vi "Read LakeShore Settings.vi"(8 "error in (no error)":errorcluster, 11 "VISA resource name":refnum<visa-resource-name>) -> (0 "error out":errorcluster, 1 "Heater level":dbl, 2 "Heater mode":T1(ring), 3 "VISA resource name out":refnum<visa-resource-name>, 4 "PID":cluster{"P":dbl, "I":dbl, "D":dbl}, 5 "Hater range":dbl, 7 "Set point":dbl)   [LabVIEW 2015]
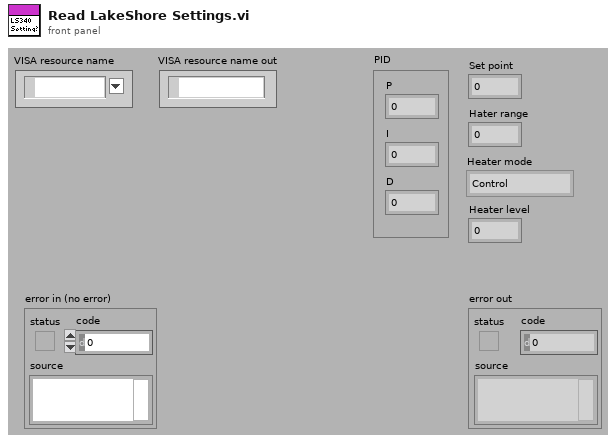
[diagram p1: front panel]
types:
  T1 = enum16{"Control", "Monitor", "Manual Heat", "Controller is in OFF mode", "Autotune is in progress"}
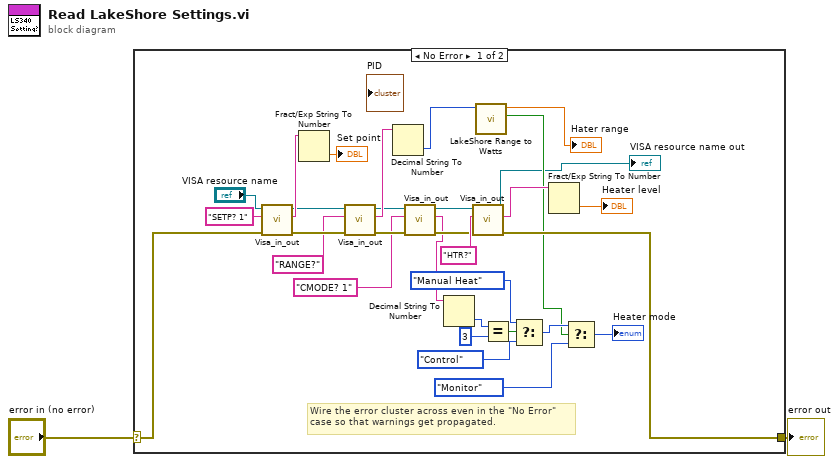
[diagram p0: block diagram]
diagram:
  n1 = case shown="No Error" "error in (no error)" {
    selector: "error in (no error)" -> [w4 w34]
    tunnel: [w17 w34] -> w1
    frame No Error {
      # "Wire the error cluster across even in the \"No Error\"\ncase so that warnings get propagated."
      n2 = call "Visa_in_out.vi"("error in (no error)"=w4, "write buffer"="SETP? 1", "VISA resource name"="VISA resource name") -> ("error out"=w30:errorcluster, "read buffer"=w32:string, "VISA resource name out"=w29:refnum<visa-resource-name>)  [unwired: 1 in, 5 out]
      n3 = Fract/Exp String To Number(string=w32) -> (number=→"Set point":dbl)  [unwired: 4 out]
      n4 = call "Visa_in_out.vi"("error in (no error)"=w30, "write buffer"="RANGE?", "VISA resource name"=w29) -> ("error out"=w19:errorcluster, "read buffer"=w27:string, "VISA resource name out"=w21:refnum<visa-resource-name>)  [unwired: 1 in, 5 out]
      n5 = Decimal String To Number(string=w27) -> (number=w26:i32)  [unwired: 3 out]
      n6 = call "Visa_in_out.vi"("error in (no error)"=w19, "write buffer"="CMODE? 1", "VISA resource name"=w21) -> ("error out"=w18:errorcluster, "read buffer"=w15:string, "VISA resource name out"=w20:refnum<visa-resource-name>)  [unwired: 1 in, 5 out]
      n7 = Decimal String To Number(string=w15) -> (number=w14:i32)  [unwired: 3 out]
      n8 = call "Visa_in_out.vi"("error in (no error)"=w18, "write buffer"="HTR?", "VISA resource name"=w20) -> ("error out"=w17:errorcluster, "read buffer"=w23:string, "VISA resource name out"=→"VISA resource name out":refnum<visa-resource-name>)  [unwired: 1 in, 5 out]
      n9 = call "LakeShore Range to Watts.vi"("Integer range"=w26) -> ("Heater off"=w10:bool, "Watts"=→"Hater range":dbl)  [unwired: 9 in]
      n10 = Equal?(x=w14, y=3) -> (x = y?=w12:bool)
      n11 = Select(t=T1."Manual Heat" ("Heater mode"), s=w12, f=T1."Control" ("Heater mode")) -> (s? t:f=w11:T1)
      n12 = Fract/Exp String To Number(string=w23) -> (number=→"Heater level":dbl)  [unwired: 4 out]
      n13 = Select(t=w11, s=w10, f=T1."Monitor" ("Heater mode")) -> (s? t:f=→"Heater mode":T1)
    }
    frame Error {
    }
  }
  "error out" <- w1
